vi "Data Get Shape.vi"(8 "error in (no error)":errorcluster, 11 "Data DVR in":refnum<data-value>) -> (0 "error out":errorcluster, 2 "Shape out":i32[](array[numeric]), 3 "Data DVR out":refnum<data-value>)   [LabVIEW 2012, in "MDSplus.lvlib"]
doc: "Gets the array dimensions as an integer array. It is implemented at this class level by computing TDI expression SHAPE(this). If shape fails an exception is generated."
uses:
  <vilib>/MDSplus/Library/MDSplus.lvlib
  <vilib>/MDSplus/Classes/Data_Class/Data.lvclass
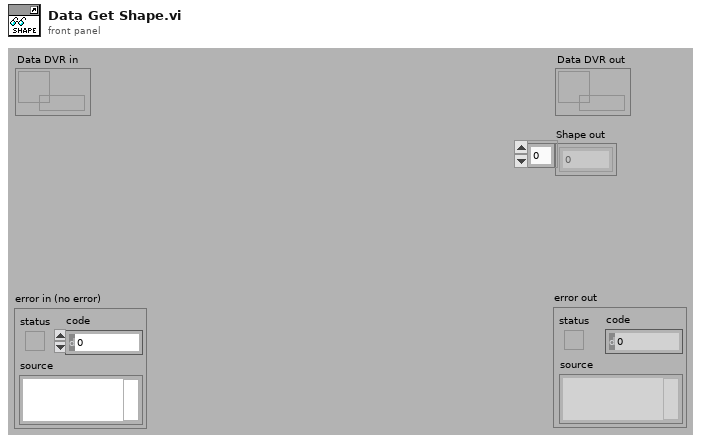
[diagram p1: front panel]
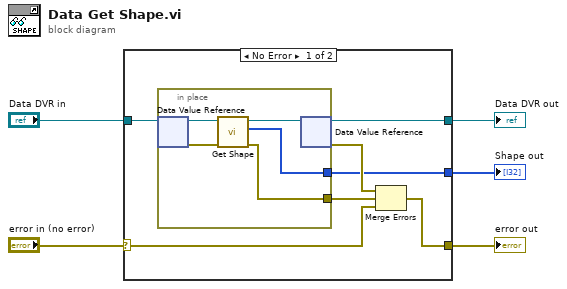
[diagram p0: block diagram]
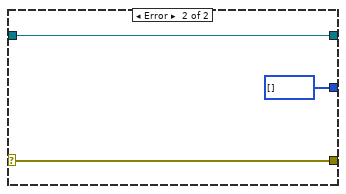
[diagram p2: hidden frame]
diagram:
  n1 = case shown="No Error" "error in (no error)" {
    selector: "error in (no error)" -> [w10 w20]
    tunnel: "Data DVR in" -> [w12 w19]
    tunnel: [w8 w20] -> w5
    tunnel: [w7 w19] -> w2
    tunnel: [w6 i32[] [] ("SGL array out")] -> w1
    frame No Error {
      n2 = in-place {
        in-place-border: [w15] -> w11
        in-place-border: [w13] -> w6
        n3 = in-place-dvr #1(w12) -> (w17:refnum<class "Data.lvclass">, w14:errorcluster)
        n4 = call-dynamic "Get Shape.vi"("error in (no error)"=w14, "Data in"=w17) -> ("error out"=w15:errorcluster, "Shape out"=w13:i32[], "Data out"=w16:refnum<class "Data.lvclass">)  [unwired: 7 in]
        n5 = in-place-dvr #1(w16) -> (w7:refnum<data-value>, w9:errorcluster)
      }
      n6 = Merge Errors(w9, w11, w10) -> (w8:errorcluster)
    }
    frame Error {
    }
  }
  "error out" <- w5
  "Data DVR out" <- w2
  "Shape out" <- w1
